vi "Convert Message Events.vi"(4 "Local Events":T1[](array[typedef])) -> (7 "Payload":u8[](array[numeric]) format="%.0x")   [LabVIEW 2020, in "Volatus.lvlib" / "Event Reporter Module.lvclass"]
uses:
  Event Reporter Module.lvclass
  Event Reporter Module.lvclass/Event Reporter Module.ctl
  messages/Error/Data.ctl
  messages/Error/Error.lvlib
  messages/EventLevel/Enumeration.ctl
  messages/EventLevel/EventLevel.lvlib
  messages/Event/Data.ctl
  messages/Event/Event.lvlib
  lv-vecto/Vecto/Vecto.lvlib
  messages/Events/Events.lvlib
  Event Level.ctl
  Volatus.lvlib
  Event.ctl
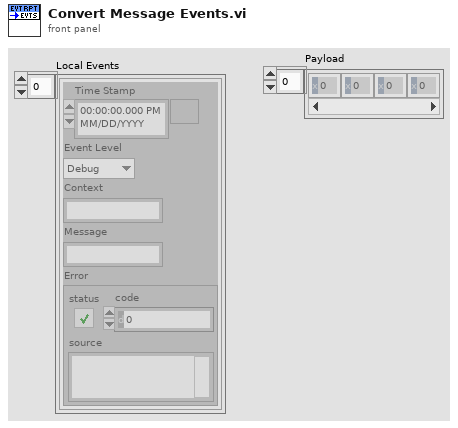
[diagram p1: front panel]
types:
  T1 = typedef "Volatus.lvlib/Event.ctl" = cluster{"Time Stamp":timestamp, "Event Level":T2, "Context":string, "Message":string, "Error":errorcluster}
  T2 = typedef "Volatus.lvlib/Event Level.ctl" = enum16{"Debug", "Info", "Warning", "Error"}
  T3 = typedef "Event.lvlib/Data.ctl" = cluster{"timestamp":i64, "level":T4, "context":string, "message":string, "error":T5}
  T4 = typedef "EventLevel.lvlib/Enumeration.ctl" = enum16{"EVENTLEVEL_UNKNOWN", "EVENTLEVEL_DEBUG", "EVENTLEVEL_INFO", "EVENTLEVEL_WARNING", "EVENTLEVEL_ERROR"}
  T5 = typedef "Error.lvlib/Data.ctl" = errorcluster
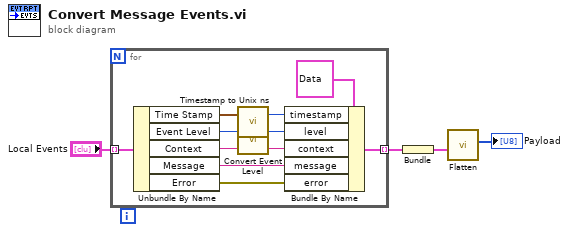
[diagram p0: block diagram]
diagram:
  n1 = for {
    tunnel: "Local Events" -> [w14] mode=indexing
    tunnel: [w5] -> w3 mode=indexing
    n2 = Unbundle By Name(w14) -> ("Time Stamp"=w13:timestamp, "Event Level"=w12:T2, "Context"=w8:string, "Message"=w9:string, "Error"=w10:errorcluster)
    n3 = call "Timestamp to Unix ns.vi"("Time Stamp"=w13) -> ("unix ns"=w6:i64)  [unwired: 2 in]
    n4 = call "Convert Event Level.vi"("Event Level"=w12) -> ("Enumeration"=w7:T4)  [unwired: 6 in]
    n5 = Bundle By Name(cluster=T3 {"timestamp"=0, "level"=enum."EVENTLEVEL_UNKNOWN", "context"="", "message"="", "error"={"status"=FALSE, "code"=0, "source"=""}}, "timestamp"=w6, "level"=w7, "context"=w8, "message"=w9, "error"=w10) -> (w5:T3)
  }
  n6 = Bundle(w3) -> (w2:cluster{T3[]})  [unwired: 1 in]
  n7 = call "Flatten.vi"("Data"=w2) -> ("Buffer"=→"Payload":u8[])  [unwired: 9 in, 1 out]
